vi "Light to Nuetral.vi"(8 "error in (no error)":errorcluster, 11 "Contestant in":refnum<class "Contestant.lvclass">) -> (0 "error out":errorcluster, 3 "Contestant out":refnum<class "Contestant.lvclass">)   [LabVIEW 2024, in "Contestant.lvlib" / "Contestant.lvclass"]
uses:
  Contestant.lvclass
  Contestant.lvclass/Contestant.ctl
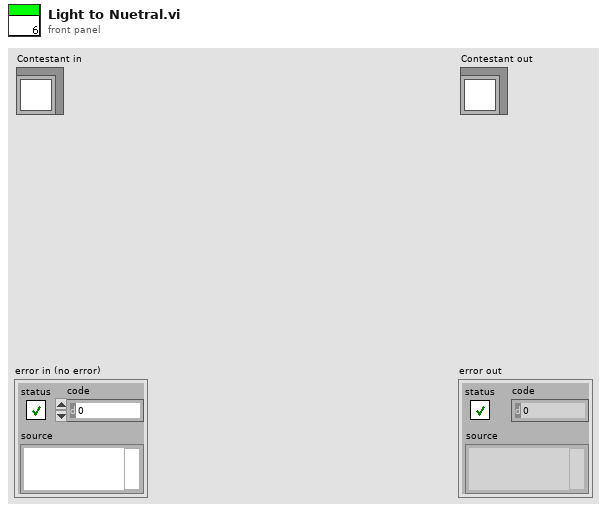
[diagram p1: front panel]
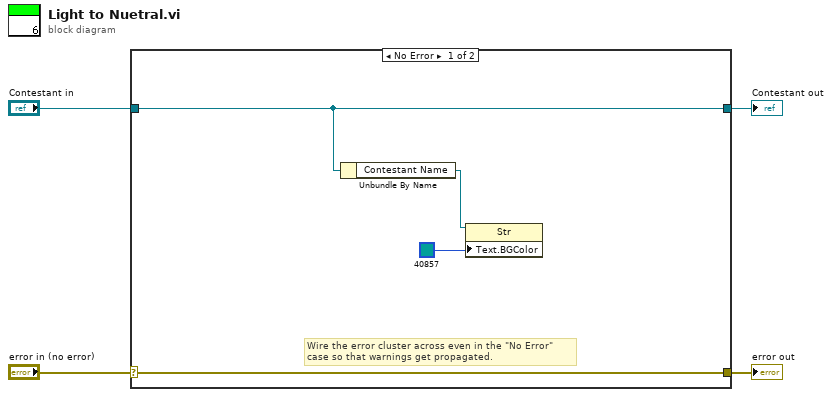
[diagram p0: block diagram]
diagram:
  n1 = case shown="No Error" "error in (no error)" {
    selector: "error in (no error)" -> [w8 w10]
    tunnel: [w8 w10] -> w3
    tunnel: [w5 w9] -> w1
    tunnel: "Contestant in" -> [w5 w9]
    frame No Error {
      # "Wire the error cluster across even in the \"No Error\"\ncase so that warnings get propagated."
      n2 = Unbundle By Name(w5) -> ("Contestant Name"=w6:refnum<vi>)
      n3 = property on="Property Node" class="Str"(reference=w6, "Text.BGColor"=u32 40857 ("Text.Text Colors:BG Color")) -> ()  [unwired: 1 in, 2 out]
    }
    frame Error {
    }
  }
  "error out" <- w3
  "Contestant out" <- w1
